vi "Unit String.vi"(8 "error in (no error)":errorcluster, 11 "Channel in":refnum<class "Channel.lvclass">) -> (0 "error out":errorcluster, 2 "Unit String":string, 3 "Channel out":refnum<class "Channel.lvclass">)   [LabVIEW 2020, in "VolatusConfig.lvlib" / "Channel.lvclass"]
uses:
  Channel.lvclass
  Channel.lvclass/Channel.ctl
  VolatusConfigElement/VolatusConfigElement.lvclass
  lv-cdm/CDM-Config/Config Element/Config Element.lvclass
  C:/dev/lv20CE/relink/lv-volatus/VolatusConfig/VolatusConfigElement/VolatusConfigElement.lvclass
  C:/dev/lv20CE/relink/lv-volatus/VolatusConfig/Channel/Channel.lvclass
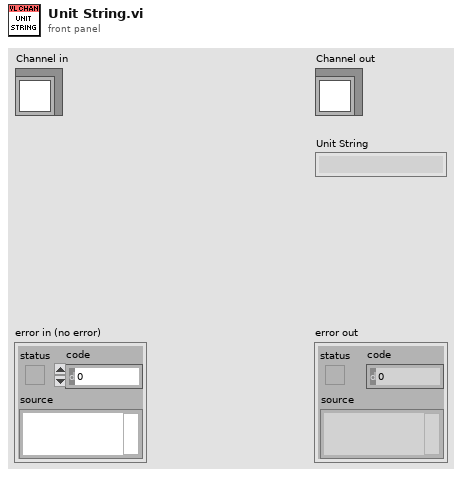
[diagram p1: front panel]
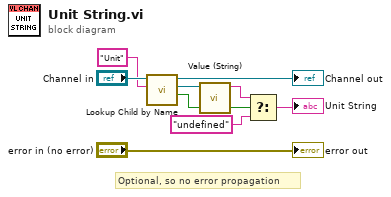
[diagram p0: block diagram]
diagram:
  # "Optional, so no error propagation"
  n1 = call "Lookup Child by Name.vi"("Child Name"="Unit", "VolatusConfigElement in"="Channel in") -> ("Found"=w3:bool, "Child"=w6:refnum<class "Config Element.lvclass">, "VolatusConfigElement out"=→"Channel out":refnum<class "Channel.lvclass">)  [unwired: 6 in, 1 out]
  n2 = call "Value (String).vi"("Config Element in"=w6) -> ("String Value"=w4:string)  [unwired: 9 in, 1 out]
  n3 = Select(t=w4, s=w3, f="undefined") -> (s? t:f=→"Unit String":string)
  "error out" <- "error in (no error)"
